vi "Remove LineFeed Constant.vi"(11 "1D String Array in":string[](array[string])) -> (3 "1D String Array out":string[](array[string]))   [LabVIEW 2019]
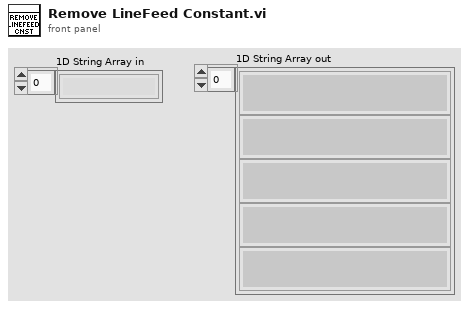
[diagram p1: front panel]
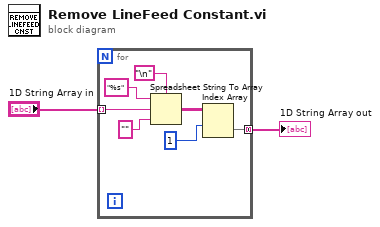
[diagram p0: block diagram]
diagram:
  n1 = for {
    tunnel: "1D String Array in" -> [w8] mode=indexing
    tunnel: [w5] -> w1 mode=concatenating
    n2 = Spreadsheet String To Array(delimiter (Tab)="\n", format string="%s", spreadsheet string=w8, array type (2D Dbl)="" ("format string")) -> (array=w4:string[][])
    n3 = Index Array(array=w4, index (row)=1 ("disabled index (col)")) -> (element=w5:string[])  [unwired: 1 in]
  }
  "1D String Array out" <- w1
